vi "MulMean.vi"(8 "IN 4":dbl[](array[numeric]) caption="X" format="%0.2f", 9 "IN 3":dbl[](array[numeric]) caption="X" format="%0.2f", 10 "IN 2":dbl[](array[numeric]) caption="X" format="%0.2f", 11 "IN 1":dbl[](array[numeric]) caption="X" format="%0.2f") -> (0 "mean 4":dbl caption="均值" format="%0.2f", 1 "mean 3":dbl caption="均值" format="%0.2f", 2 "mean 2":dbl caption="均值" format="%0.2f", 3 "mean 1":dbl caption="均值" format="%0.2f")   [LabVIEW 2024]
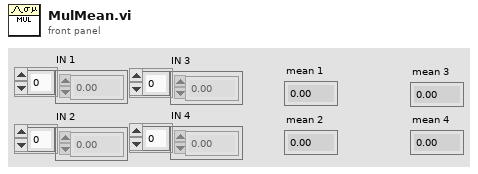
[diagram p1: front panel]
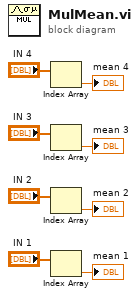
[diagram p0: block diagram]
diagram:
  n1 = Index Array(array="IN 4") -> (element=→"mean 4":dbl)  [unwired: 1 in]
  n2 = Index Array(array="IN 3") -> (element=→"mean 3":dbl)  [unwired: 1 in]
  n3 = Index Array(array="IN 2") -> (element=→"mean 2":dbl)  [unwired: 1 in]
  n4 = Index Array(array="IN 1") -> (element=→"mean 1":dbl)  [unwired: 1 in]
